vi "_updateConnectionPid.vi"(8 "error in (no error)":errorcluster, 9 "PID":i64, 10 "GUID":string, 11 "tWorkerController in":refnum<class "tWorkerController.lvclass">) -> (0 "error out":errorcluster, 3 "tWorkerController out":refnum<class "tWorkerController.lvclass">)   [LabVIEW 2013, in "tWorkerController.lvlib" / "tWorkerController.lvclass"]
uses:
  tWorkerController.lvclass
  tWorkerController.lvclass/tWorkerController.ctl
  _status.ctl
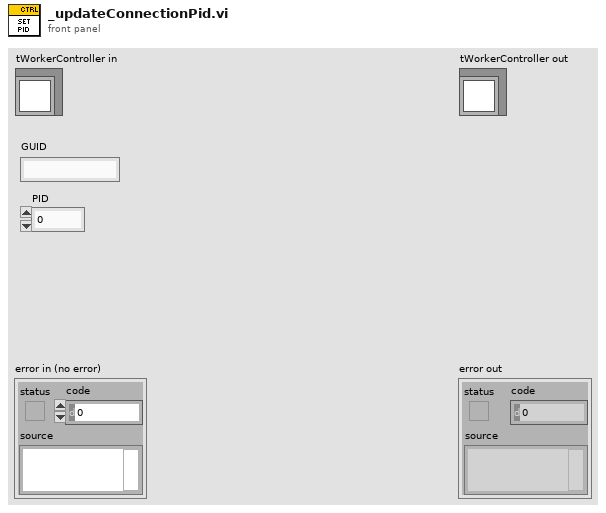
[diagram p1: front panel]
types:
  T1 = typedef "tWorkerController.lvlib/tWorkerController.lvclass/_status.ctl" = enum16{"Problem Launching Worker", "Worker Not Found", "Test Not In Library", "Connection Not Found"}
  T2 = typedef "tWorkerController.lvlib/tWorkerController.lvclass/_tcpConnection.ctl" = cluster{"GUID":string, "Connection Queue":refnum<class "Message Enqueuer.lvclass">, "PID":i64}
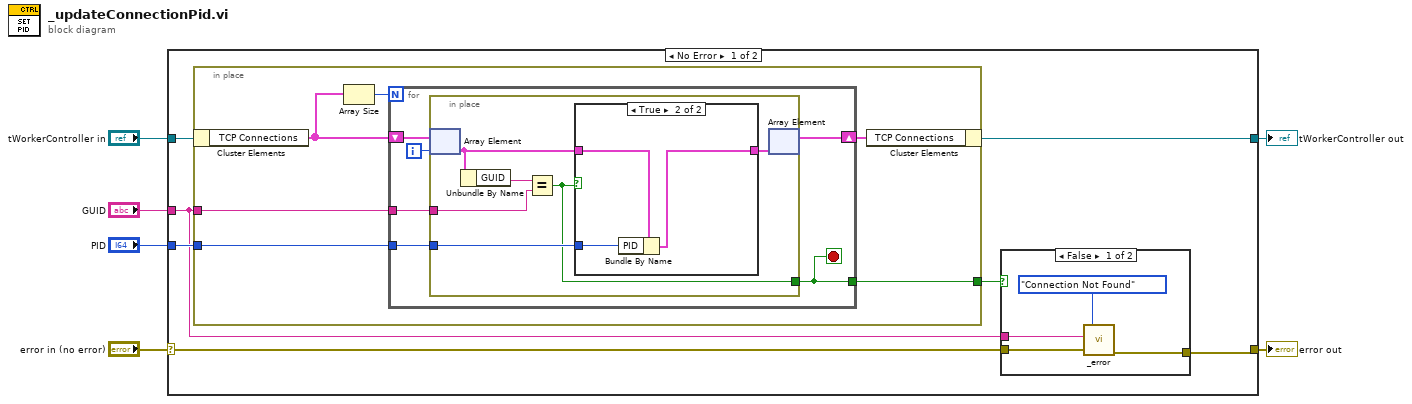
[diagram p0: block diagram]
diagram:
  n1 = case shown="No Error" "error in (no error)" {
    selector: "error in (no error)" -> [w10 w42]
    tunnel: [w8 w42] -> w5
    tunnel: [w7 w41] -> w3
    tunnel: "tWorkerController in" -> [w13 w41]
    tunnel: "GUID" -> [w9 _]
    tunnel: "PID" -> [w12 _]
    frame No Error {
      n2 = in-place {
        in-place-border: w9 -> [w21]
        in-place-border: w12 -> [w20]
        in-place-border: [w19] -> w11
        n3 = in-place-cluster #1(w13) -> ("TCP Connections"=w23:T2[])
        n4 = Array Size(array=w23) -> (size(s)=w24:i32)
        n5 = for {
          N: w24 -> [_]
          shift-right: [w26] -> w22
          shift-left: w23 -> [w30]
          tunnel: w21 -> [w28]
          tunnel: w20 -> [w27]
          tunnel: [w25] -> w19
          i -> [w29]
          stop <- w25 stop-if-true
          n6 = in-place {
            in-place-border: w28 -> [w35]
            in-place-border: w27 -> [w33]
            in-place-border: [w31] -> w25
            n7 = in-place-array #2(w30, w29) -> (w34:T2)
            n8 = Unbundle By Name(w34) -> ("GUID"=w36:string)
            n9 = Equal?(x=w36, y=w35) -> (x = y?=w31:bool)
            n10 = case shown="True" w31 {
              tunnel: w34 -> [w37 w40]
              tunnel: w33 -> [_ w39]
              tunnel: [w37 w38] -> w32
              frame False {
              }
              frame True {
                n11 = Bundle By Name(cluster=w40, "PID"=w39) -> (w38:T2)
              }
            }
            n12 = in-place-array #2(w32) -> (w26:T2[])  [unwired: 1 out]
          }
        }
        n13 = in-place-cluster #1("TCP Connections"=w22) -> (w7:refnum<class "tWorkerController.lvclass">)
      }
      n14 = case shown="False" w11 {
        tunnel: w10 -> [w17 w18]
        tunnel: w9 -> [w15 _]
        tunnel: [w14 w18] -> w8
        frame False {
          n15 = call "_error.vi"("error in (no error)"=w17, "Additional message"=w15, "Status"=_status."Connection Not Found") -> ("error out"=w14:errorcluster)  [unwired: 8 in]
        }
        frame True {
        }
      }
    }
    frame Error {
    }
  }
  "error out" <- w5
  "tWorkerController out" <- w3
